vi "moveMotor.vi"(2 "移动位置":dbl, 3 "步进电机串口":refnum<visa-resource-name>) -> (0 "串口返回结果":string, 1 "步进电机串口返回":refnum<visa-resource-name>)   [LabVIEW 2018]
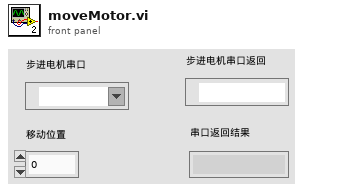
[diagram p1: front panel]
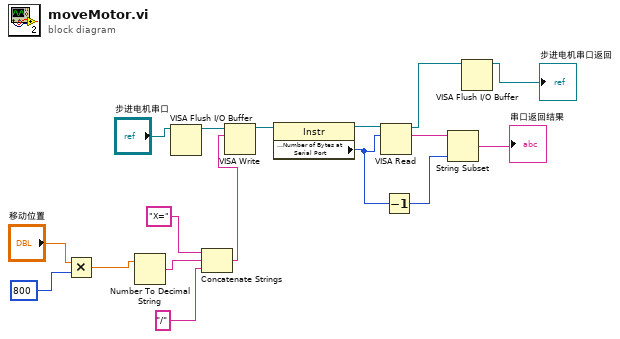
[diagram p0: block diagram]
diagram:
  n1 = Multiply(x="移动位置", y=800) -> (x*y=w9:dbl)
  n2 = Number To Decimal String(number=w9) -> (decimal integer string=w7:string)  [unwired: 1 in]
  n3 = VISA Flush I/O Buffer(VISA resource name="步进电机串口") -> (VISA resource name out=w1:refnum<visa-resource-name>)  [unwired: 2 in, 1 out]
  n4 = Concatenate Strings("X=", w7, "/") -> (w5:string)
  n5 = VISA Write(VISA resource name=w1, write buffer=w5) -> (VISA resource name out=w16:refnum<visa-resource-name>)  [unwired: 1 in, 2 out]
  n6 = property class="Instr"(reference=w16) -> (reference out=w17:refnum<visa-resource-name>, "Serial Settings:Number of Bytes at Serial Port"=w13:u32)  [unwired: 1 in, 1 out]
  n7 = VISA Read(VISA resource name=w17, byte count=w13) -> (VISA resource name out=w4:refnum<visa-resource-name>, read buffer=w15:string)  [unwired: 1 in, 2 out]
  n8 = Decrement(x=w13) -> (x-1=w12:u32)
  n9 = String Subset(string=w15, length (rest)=w12) -> (substring=→"串口返回结果":string)  [unwired: 1 in]
  n10 = VISA Flush I/O Buffer(VISA resource name=w4) -> (VISA resource name out=→"步进电机串口返回":refnum<visa-resource-name>)  [unwired: 2 in, 1 out]
